vi "StanleyMethod.vi"(2 "v(Velocity)m/s":dbl, 3 "e(Cross-Track Err)m/s":dbl, 4 "k(Gain)":dbl, 5 "¥÷(Heading Err)radian":dbl) -> (0 "ヤ(OutputSteer)radian":dbl, 1 "ヤ(OutputSteer)degrees":dbl)   [LabVIEW 2024]
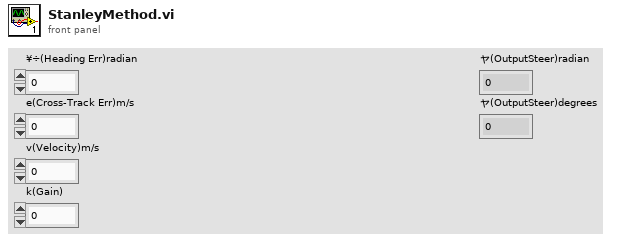
[diagram p1: front panel]
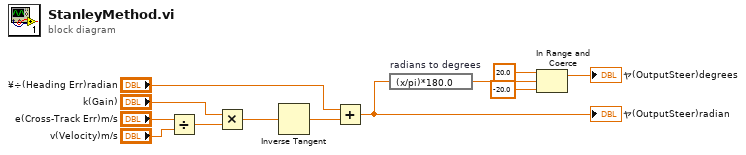
[diagram p0: block diagram]
diagram:
  n1 = Divide(x="e(Cross-Track Err)m/s", y="v(Velocity)m/s") -> (x/y=w9:dbl)
  n2 = Multiply(x="k(Gain)", y=w9) -> (x*y=w10:dbl)
  n3 = Inverse Tangent(1:w10) -> (0:w11:dbl)
  n4 = Add(x="¥÷(Heading Err)radian", y=w11) -> (x+y=w5:dbl)
  "ヤ(OutputSteer)radian" <- w5
  n5 = expression code="(x/pi)*180.0" "radians to degrees"(w5) -> (w1:dbl)
  n6 = In Range and Coerce(upper limit=20.0, x=w1, lower limit=-20.0) -> (coerced(x)=→"ヤ(OutputSteer)degrees":dbl)  [unwired: 1 out]
